vi "onDisconnection.vi"(8 "error in (no error)":errorcluster, 11 "Connection.TCP":refnum<class "Connection.Collection.lvclass">) -> (0 "error out":errorcluster, 3 "No Connection":refnum<class "Connection.Collection.lvclass">)   [LabVIEW 2013, in "Connection_GOSPL.lvlib" / "Connection.Collection.lvclass"]
uses:
  Connection.Collection.lvclass
  Connection.Collection.lvclass/Connection.Collection.ctl
  Connection/Connection.lvclass
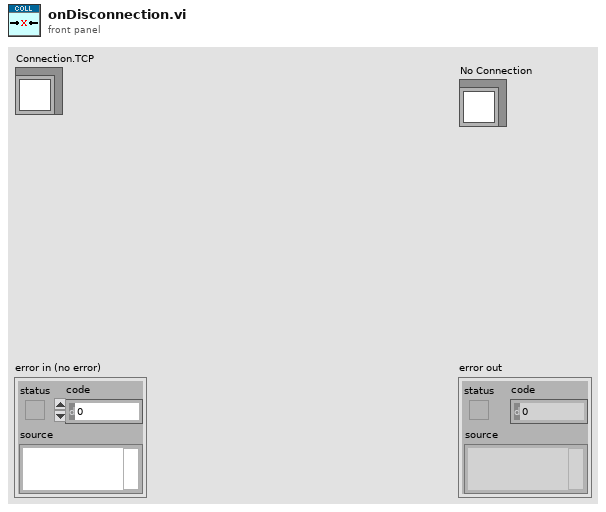
[diagram p1: front panel]
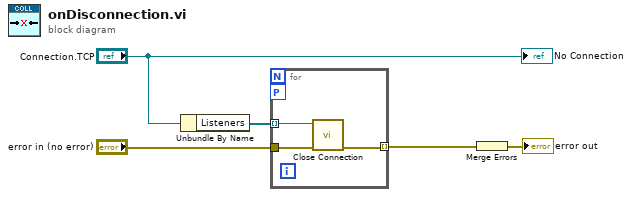
[diagram p0: block diagram]
diagram:
  n1 = Unbundle By Name("Connection.TCP") -> ("Listeners"=w2:refnum<class "Connection.lvclass">[])
  n2 = for {
    tunnel: "error in (no error)" -> [w7]
    tunnel: [w6] -> w4 mode=indexing
    tunnel: w2 -> [w8] mode=indexing
    workers-P: _ -> [_]
    n3 = call "Close Connection.vi"("error in (no error)"=w7, "Connection in"=w8) -> ("error out"=w6:errorcluster)  [unwired: 8 in, 1 out]
  }
  n4 = Merge Errors(w4) -> (→"error out":errorcluster)
  "No Connection" <- "Connection.TCP"
